vi "Clear All.vi"(8 "error in (no error)":errorcluster, 11 "Canvas in":refnum<class "Canvas.lvclass">) -> (0 "error out":errorcluster, 3 "Canvas out":refnum<class "Canvas.lvclass">)   [LabVIEW 2015, in "Canvas.lvclass"]
uses:
  Canvas.lvclass
  Graphic/Graphic.lvclass
  Canvas.lvclass/Canvas.ctl
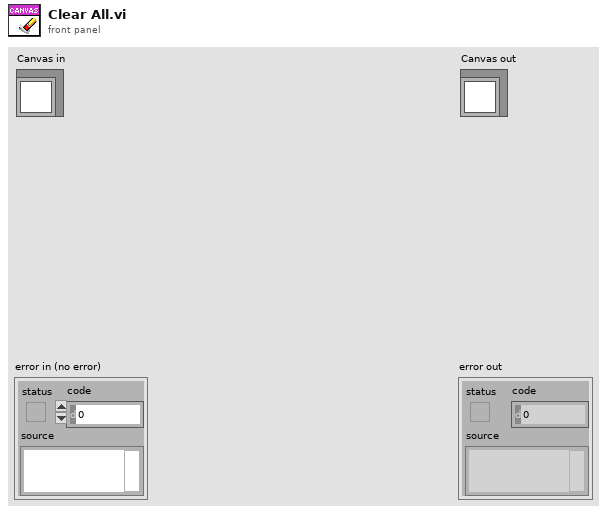
[diagram p1: front panel]
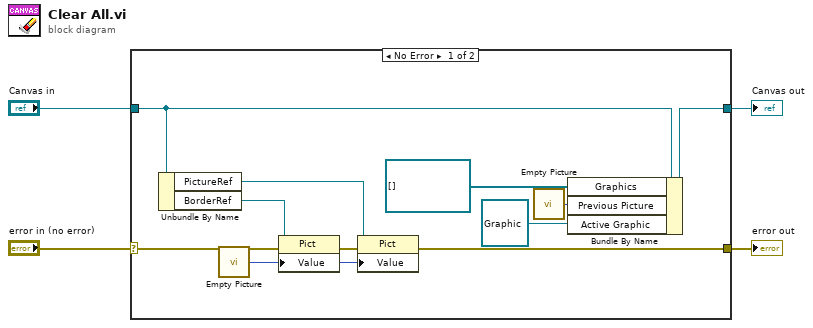
[diagram p0: block diagram]
diagram:
  n1 = case shown="No Error" "error in (no error)" {
    selector: "error in (no error)" -> [w6 w17]
    tunnel: [w7 w17] -> w3
    tunnel: [w11 w16] -> w1
    tunnel: "Canvas in" -> [w15 w16]
    frame No Error {
      n2 = Unbundle By Name(w15) -> ("PictureRef"=w12:refnum<vi>, "BorderRef"=w14:refnum<vi>)
      n3 = call "Empty Picture"() -> ("empty picture"=w5:picture)
      n4 = property class="Pict"(reference=w14, error in=w6, "Value"=w5) -> (error out=w13:errorcluster)  [unwired: 1 out]
      n5 = property class="Pict"(reference=w12, error in=w13, "Value"=w5) -> (error out=w7:errorcluster)  [unwired: 1 out]
      n6 = call "Empty Picture"() -> ("empty picture"=w8:picture)
      n7 = Bundle By Name(cluster=w15, "Graphics"=refnum<class "Graphic.lvclass">[] [], "Previous Picture"=w8, "Active Graphic"=refnum<class "Graphic.lvclass"> refnum) -> (w11:refnum<class "Canvas.lvclass">)
    }
    frame Error {
    }
  }
  "error out" <- w3
  "Canvas out" <- w1
